vi "getPulseDurationAcq.vi"(8 "error in (no error)":errorcluster, 11 "Acquisition in":refnum<class "Acquisition.lvclass">) -> (0 "error out":errorcluster, 2 "Pulse Duration":dbl[](array[numeric]), 3 "Acquisition out":refnum<class "Acquisition.lvclass">)   [LabVIEW 2014]
uses:
  Acquisition.lvclass
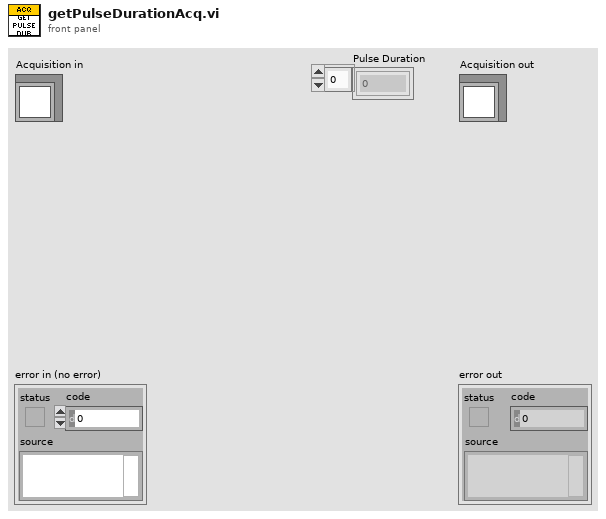
[diagram p1: front panel]
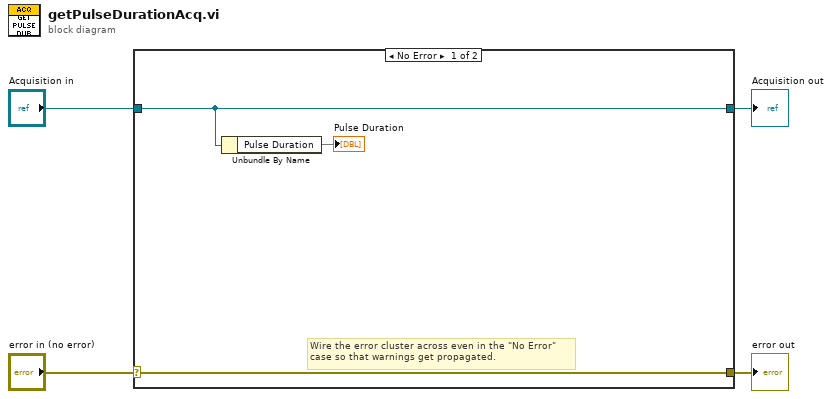
[diagram p0: block diagram]
diagram:
  n1 = case shown="No Error" "error in (no error)" {
    selector: "error in (no error)" -> [w7 w9]
    tunnel: [w7 w9] -> w3
    tunnel: [w6 w8] -> w1
    tunnel: "Acquisition in" -> [w6 w8]
    frame No Error {
      # "Wire the error cluster across even in the \"No Error\"\ncase so that warnings get propagated."
      n2 = Unbundle By Name(w6) -> ("Pulse Duration"=→"Pulse Duration")
    }
    frame Error {
    }
  }
  "error out" <- w3
  "Acquisition out" <- w1
